vi "WriteStimulus.vi"(8 "error in (no error)":errorcluster, 10 "Stimulus":sgl[][](array[numeric]), 11 "StimulusObject in":refnum<class "StimulusObject.lvclass">) -> (0 "error out":errorcluster, 3 "StimulusObject out":refnum<class "StimulusObject.lvclass">)   [LabVIEW 2019, in "StimulusObject.lvclass"]
uses:
  StimulusObject.lvclass
  StimulusObject.lvclass/StimulusObject.ctl
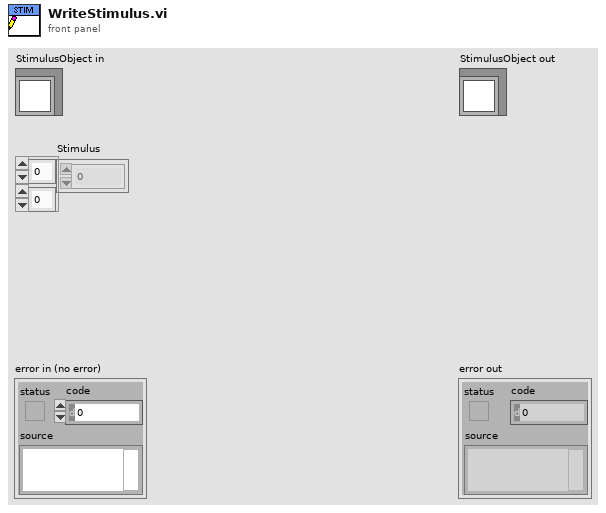
[diagram p1: front panel]
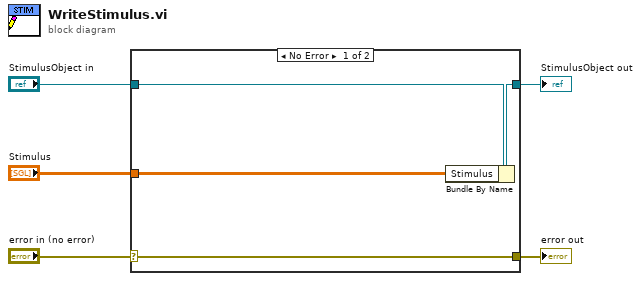
[diagram p0: block diagram]
diagram:
  n1 = case shown="No Error" "error in (no error)" {
    selector: "error in (no error)" -> [w9 w10]
    tunnel: [w9 w10] -> w4
    tunnel: [w7 w11] -> w2
    tunnel: "StimulusObject in" -> [w8 w11]
    tunnel: "Stimulus" -> [w6 _]
    frame No Error {
      n2 = Bundle By Name(cluster=w8, "Stimulus"=w6) -> (w7:refnum<class "StimulusObject.lvclass">)
    }
    frame Error {
    }
  }
  "error out" <- w4
  "StimulusObject out" <- w2
